vi "HW1_0716007_1011.vi"() -> ()   [LabVIEW 2018]
panel:
  out "Boolean 36":bool
  in  "Boolean 35":bool
  in  "Boolean 30":bool
  out "Boolean 29":bool
  out "Boolean 28":bool
  out "Boolean 27":bool
  out "Boolean 26":bool
  out "Boolean 25":bool
  out "Boolean 24":bool
  out "Boolean 23":bool
  out "Boolean 22":bool
  out "Boolean 21":bool
  out "Boolean 20":bool
  out "Boolean 19":bool
  out "Boolean 18":bool
  out "Boolean 17":bool
  out "Boolean 16":bool
  out "Boolean 15":bool
  out "Boolean 14":bool
  out "Boolean 13":bool
  out "Boolean 12":bool
  out "Boolean 11":bool
  out "Boolean 10":bool
  out "Boolean 9":bool
  out "Boolean 8":bool
  out "Boolean 7":bool
  out "Boolean 6":bool
  out "Boolean 5":bool
  out "Boolean 4":bool
  out "Boolean 3":bool
  out "Boolean 2":bool
  out "two":dbl
  out "History one":dbl
  in  "Boolean":bool
  out "Numeric":dbl
  in  "stop":bool
  out "String 2":string
  out "String":string
  in  "=":bool
  in  "Sqrt":bool
  in  "1/x":bool
  in  "/":bool
  in  "*":bool
  in  "-":bool
  in  "+":bool
  in  ".":bool
  in  "+/-":bool
  in  ")":bool
  in  "(":bool
  in  "Backspace":bool
  in  "C":bool
  in  "CE":bool
  in  "0":bool
  in  "9":bool
  in  "8":bool
  in  "7":bool
  in  "6":bool
  in  "5":bool
  in  "4":bool
  in  "3":bool
  in  "2":bool
  in  "1":bool
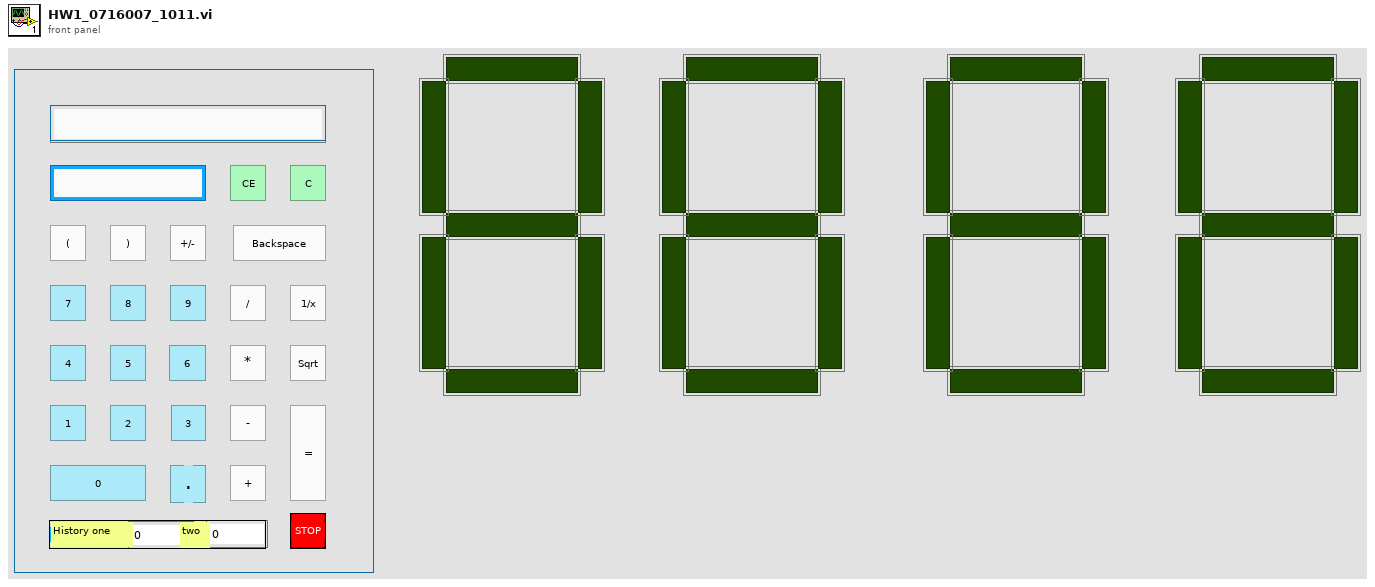
[diagram p1: front panel]
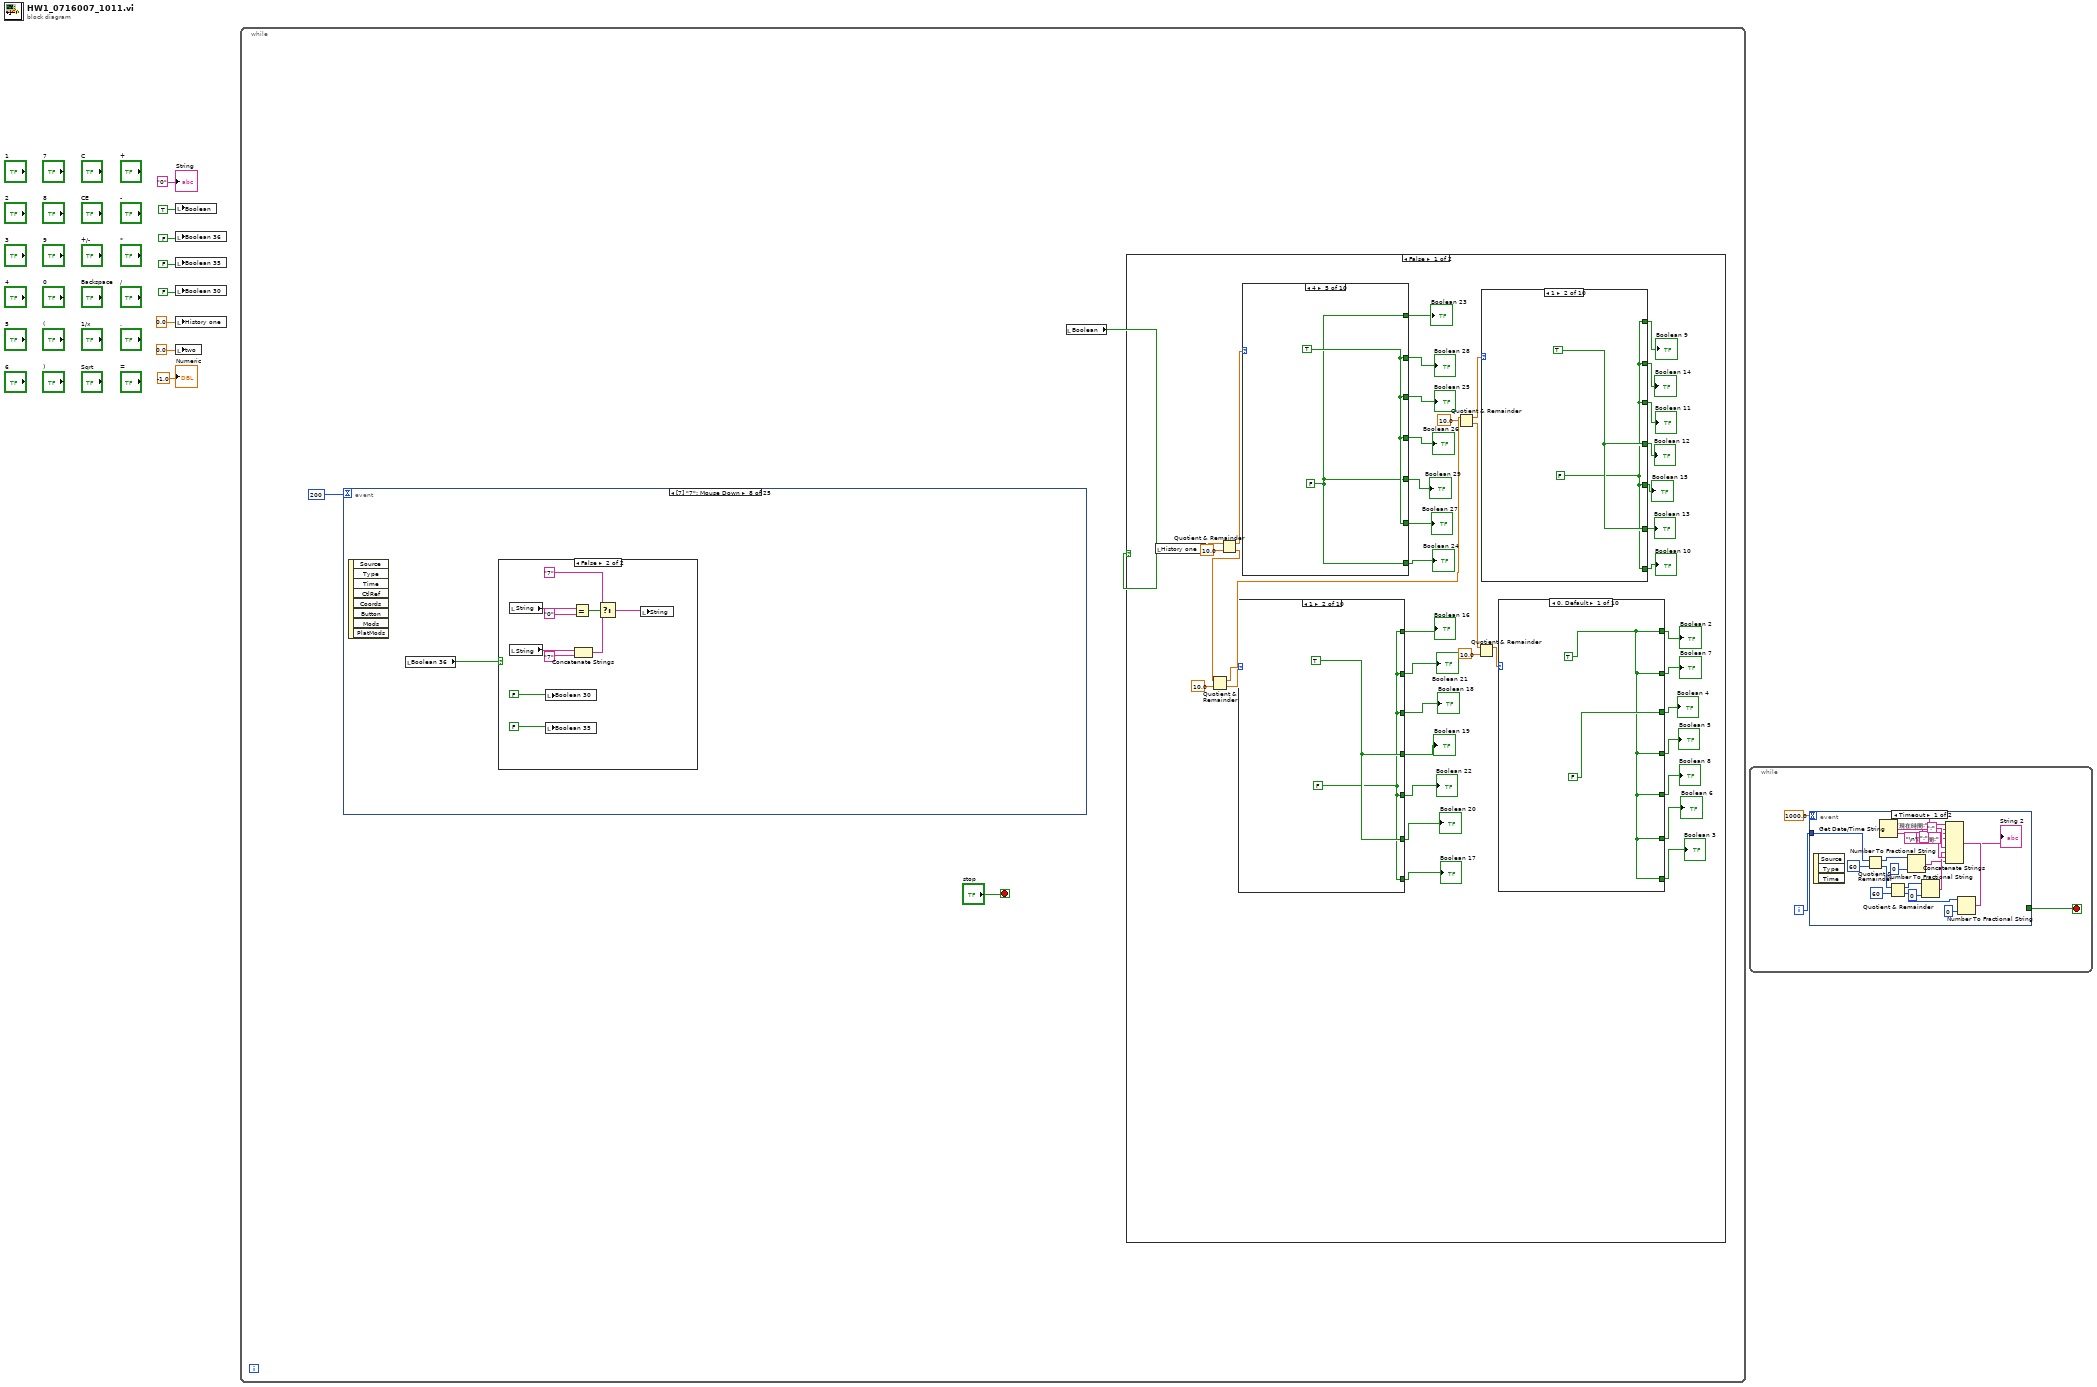
[diagram p0: block diagram]
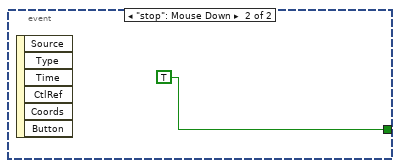
[diagram p2: hidden frame]
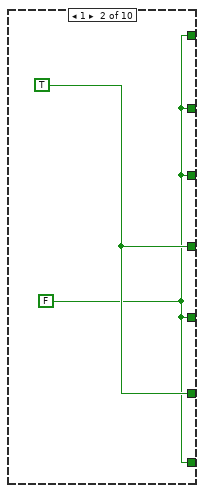
[diagram p3: hidden frame]
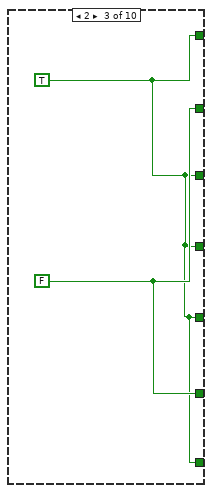
[diagram p4: hidden frame]
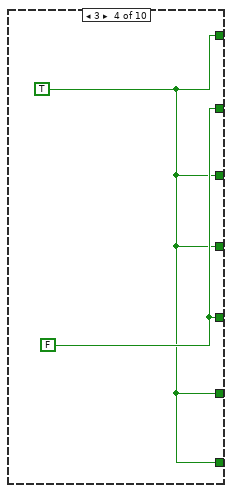
[diagram p5: hidden frame]
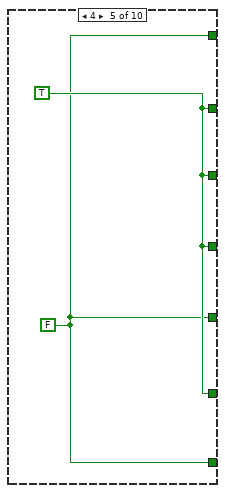
[diagram p6: hidden frame]
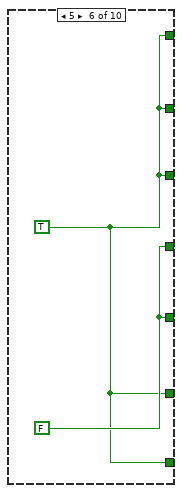
[diagram p7: hidden frame]
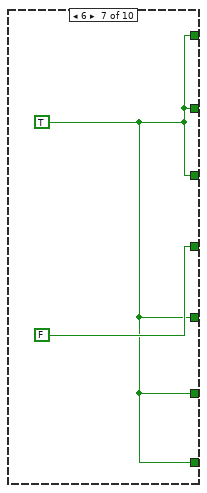
[diagram p8: hidden frame]
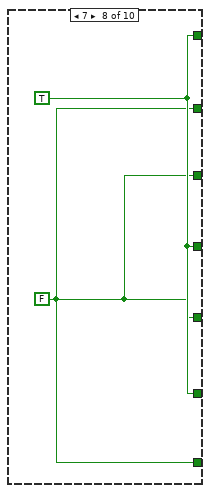
[diagram p9: hidden frame]
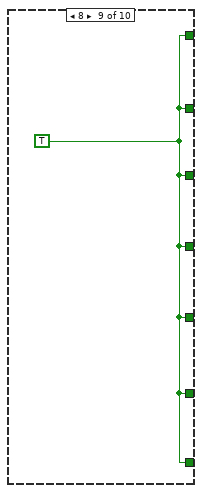
[diagram p10: hidden frame]
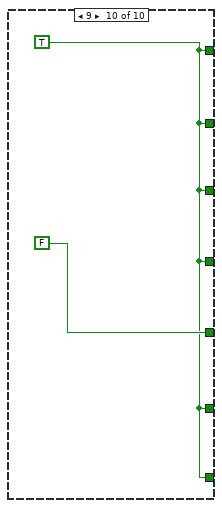
[diagram p11: hidden frame]
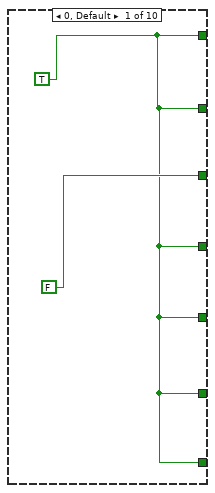
[diagram p12: hidden frame]
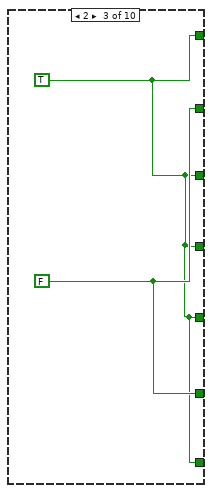
[diagram p13: hidden frame]
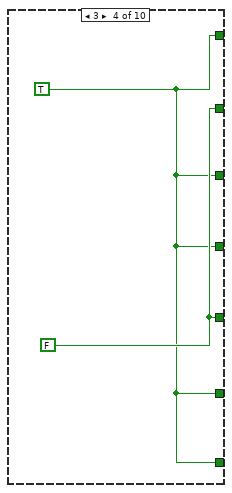
[diagram p14: hidden frame]
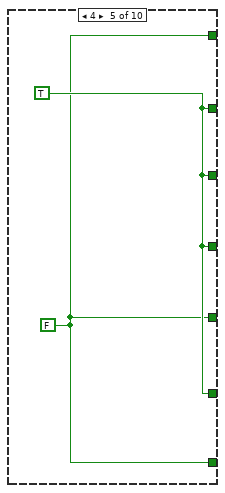
[diagram p15: hidden frame]
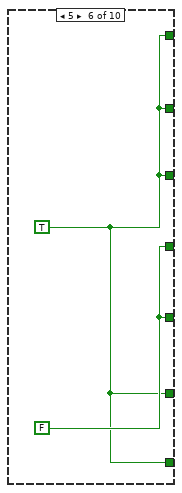
[diagram p16: hidden frame]
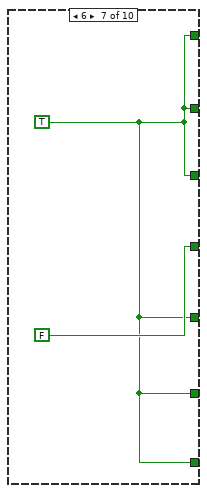
[diagram p17: hidden frame]
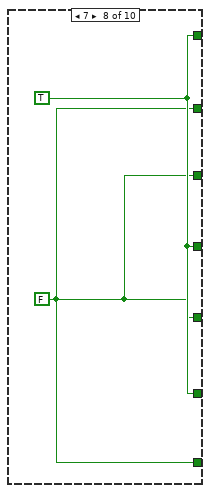
[diagram p18: hidden frame]
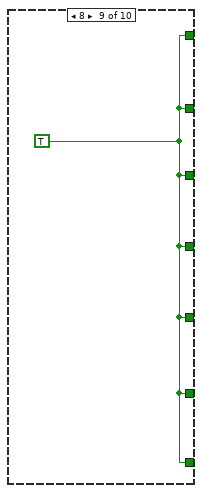
[diagram p19: hidden frame]
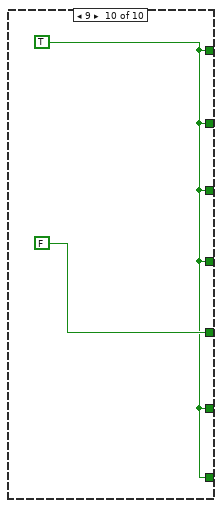
[diagram p20: hidden frame]
diagram:
  n1 = local write "Boolean"(TRUE) -> ()
  n2 = local write "Boolean 36"(FALSE ("Boolean 35")) -> ()
  n3 = local write "Boolean 35"(FALSE ("Boolean 35")) -> ()
  n4 = local write "Boolean 30"(FALSE) -> ()
  n5 = local write "History one"(0.0 ("歷史紀錄2")) -> ()
  n6 = local write "two"(0.0 ("歷史紀錄1")) -> ()
  n7 = while {
    stop <- "stop" stop-if-true
    n8 = event shown="[7] \"7\": Mouse Down" {
      selector: _ -> [_ _ _ _ _ _ _ _ _ _ _ _ _ _ _ _ _ _ _ _ _ _ _ _ _]
      dyn-events: _ -> [_ _ _ _ _ _ _ _ _ _ _ _ _ _ _ _ _ _ _ _ _ _ _ _ _]
      timeout: 200 -> [_ _ _ _ _ _ _ _ _ _ _ _ _ _ _ _ _ _ _ _ _ _ _ _ _]
      event Timeout {
        n9 = event-data() -> ()  [unwired: 1 in, 3 out]
      }
      event "1": Mouse Down {
        n10 = event-data() -> ()  [unwired: 1 in, 8 out]
        n11 = local read "Boolean 10"() -> (w244:bool)
        n12 = case shown="False" w244 {
          frame True {
            n13 = local write "String"("1" ("String")) -> ()
            n14 = local write "Boolean 36"(FALSE) -> ()
            n15 = local write "Boolean 30"(FALSE) -> ()
          }
          frame False {
            n16 = local read "String"() -> (w254:string)
            n17 = local read "String"() -> (w257:string)
            n18 = local write "Boolean 30"(FALSE) -> ()
            n19 = local write "Boolean 35"(FALSE) -> ()
            n20 = Equal?(x=w254, y="0") -> (x = y?=w255:bool)
            n21 = Concatenate Strings(w257, "1" ("string")) -> (w251:string)
            n22 = Select(t="1" ("string"), s=w255, f=w251) -> (s? t:f=w252:string)
            n23 = local write "String"(w252) -> ()
          }
        }
      }
      event "2": Mouse Down {
        n24 = event-data() -> ()  [unwired: 1 in, 8 out]
        n25 = local read "Boolean 36"() -> (w258:bool)
        n26 = case shown="False" w258 {
          frame True {
            n27 = local write "Boolean 36"(FALSE) -> ()
            n28 = local write "String"("2" ("String")) -> ()
            n29 = local write "Boolean 30"(FALSE) -> ()
          }
          frame False {
            n30 = local read "String"() -> (w266:string)
            n31 = local read "String"() -> (w268:string)
            n32 = local write "Boolean 30"(FALSE) -> ()
            n33 = local write "Boolean 35"(FALSE) -> ()
            n34 = Equal?(x=w266, y="0") -> (x = y?=w271:bool)
            n35 = Concatenate Strings(w268, "2" ("string")) -> (w270:string)
            n36 = Select(t="2", s=w271, f=w270) -> (s? t:f=w269:string)
            n37 = local write "String"(w269) -> ()
          }
        }
      }
      event "3": Mouse Down {
        n38 = event-data() -> ()  [unwired: 1 in, 8 out]
        n39 = local read "Boolean 36"() -> (w272:bool)
        n40 = case shown="False" w272 {
          frame True {
            n41 = local write "Boolean 36"(FALSE) -> ()
            n42 = local write "String"("3" ("String")) -> ()
            n43 = local write "Boolean 30"(FALSE) -> ()
          }
          frame False {
            n44 = local read "String"() -> (w280:string)
            n45 = local read "String"() -> (w282:string)
            n46 = local write "Boolean 30"(FALSE) -> ()
            n47 = local write "Boolean 35"(FALSE) -> ()
            n48 = Equal?(x=w280, y="0") -> (x = y?=w285:bool)
            n49 = Concatenate Strings(w282, "3" ("string")) -> (w284:string)
            n50 = Select(t="3", s=w285, f=w284) -> (s? t:f=w283:string)
            n51 = local write "String"(w283) -> ()
          }
        }
      }
      event "4": Mouse Down {
        n52 = event-data() -> ()  [unwired: 1 in, 8 out]
        n53 = local read "Boolean 36"() -> (w286:bool)
        n54 = case shown="False" w286 {
          frame True {
            n55 = local write "Boolean 36"(FALSE) -> ()
            n56 = local write "String"("4" ("String")) -> ()
            n57 = local write "Boolean 30"(FALSE) -> ()
          }
          frame False {
            n58 = local read "String"() -> (w294:string)
            n59 = local read "String"() -> (w296:string)
            n60 = local write "Boolean 30"(FALSE) -> ()
            n61 = local write "Boolean 35"(FALSE) -> ()
            n62 = Equal?(x=w294, y="0") -> (x = y?=w299:bool)
            n63 = Concatenate Strings(w296, "4" ("string")) -> (w298:string)
            n64 = Select(t="4", s=w299, f=w298) -> (s? t:f=w297:string)
            n65 = local write "String"(w297) -> ()
          }
        }
      }
      event "5": Mouse Down {
        n66 = event-data() -> ()  [unwired: 1 in, 8 out]
        n67 = local read "Boolean 36"() -> (w300:bool)
        n68 = case shown="False" w300 {
          frame True {
            n69 = local write "Boolean 36"(FALSE) -> ()
            n70 = local write "String"("5" ("String")) -> ()
            n71 = local write "Boolean 30"(FALSE) -> ()
          }
          frame False {
            n72 = local read "String"() -> (w308:string)
            n73 = local read "String"() -> (w310:string)
            n74 = local write "Boolean 30"(FALSE) -> ()
            n75 = local write "Boolean 35"(FALSE) -> ()
            n76 = Equal?(x=w308, y="0") -> (x = y?=w313:bool)
            n77 = Concatenate Strings(w310, "5" ("string")) -> (w312:string)
            n78 = Select(t="5", s=w313, f=w312) -> (s? t:f=w311:string)
            n79 = local write "String"(w311) -> ()
          }
        }
      }
      event "6": Mouse Down {
        n80 = event-data() -> ()  [unwired: 1 in, 8 out]
        n81 = local read "Boolean 36"() -> (w314:bool)
        n82 = case shown="False" w314 {
          frame True {
            n83 = local write "Boolean 36"(FALSE) -> ()
            n84 = local write "String"("6" ("String")) -> ()
            n85 = local write "Boolean 30"(FALSE) -> ()
          }
          frame False {
            n86 = local read "String"() -> (w322:string)
            n87 = local read "String"() -> (w324:string)
            n88 = local write "Boolean 30"(FALSE) -> ()
            n89 = local write "Boolean 35"(FALSE) -> ()
            n90 = Equal?(x=w322, y="0") -> (x = y?=w327:bool)
            n91 = Concatenate Strings(w324, "6" ("string")) -> (w326:string)
            n92 = Select(t="6", s=w327, f=w326) -> (s? t:f=w325:string)
            n93 = local write "String"(w325) -> ()
          }
        }
      }
      event "7": Mouse Down {
        n94 = event-data() -> ()  [unwired: 1 in, 8 out]
        n95 = local read "Boolean 36"() -> (w328:bool)
        n96 = case shown="False" w328 {
          frame True {
            n97 = local write "Boolean 36"(FALSE) -> ()
            n98 = local write "String"("7" ("String")) -> ()
            n99 = local write "Boolean 30"(FALSE) -> ()
          }
          frame False {
            n100 = local read "String"() -> (w336:string)
            n101 = local read "String"() -> (w338:string)
            n102 = local write "Boolean 30"(FALSE) -> ()
            n103 = local write "Boolean 35"(FALSE) -> ()
            n104 = Equal?(x=w336, y="0") -> (x = y?=w341:bool)
            n105 = Concatenate Strings(w338, "7" ("string")) -> (w340:string)
            n106 = Select(t="7", s=w341, f=w340) -> (s? t:f=w339:string)
            n107 = local write "String"(w339) -> ()
          }
        }
      }
      event "8": Mouse Down {
        n108 = event-data() -> ()  [unwired: 1 in, 8 out]
        n109 = local read "Boolean 36"() -> (w342:bool)
        n110 = case shown="True" w342 {
          frame True {
            n111 = local write "Boolean 36"(FALSE) -> ()
            n112 = local write "String"("8" ("String")) -> ()
            n113 = local write "Boolean 30"(FALSE) -> ()
          }
          frame False {
            n114 = local read "String"() -> (w350:string)
            n115 = local read "String"() -> (w352:string)
            n116 = local write "Boolean 30"(FALSE) -> ()
            n117 = local write "Boolean 35"(FALSE) -> ()
            n118 = Equal?(x=w350, y="0") -> (x = y?=w355:bool)
            n119 = Concatenate Strings(w352, "8" ("string")) -> (w354:string)
            n120 = Select(t="8", s=w355, f=w354) -> (s? t:f=w353:string)
            n121 = local write "String"(w353) -> ()
          }
        }
      }
      event "9": Mouse Down {
        n122 = event-data() -> ()  [unwired: 1 in, 8 out]
        n123 = local read "Boolean 36"() -> (w356:bool)
        n124 = case shown="True" w356 {
          frame True {
            n125 = local write "Boolean 36"(FALSE) -> ()
            n126 = local write "String"("9" ("String")) -> ()
            n127 = local write "Boolean 30"(FALSE) -> ()
          }
          frame False {
            n128 = local read "String"() -> (w364:string)
            n129 = local read "String"() -> (w366:string)
            n130 = local write "Boolean 30"(FALSE) -> ()
            n131 = local write "Boolean 35"(FALSE) -> ()
            n132 = Equal?(x=w364, y="0") -> (x = y?=w369:bool)
            n133 = Concatenate Strings(w366, "9" ("string")) -> (w368:string)
            n134 = Select(t="9", s=w369, f=w368) -> (s? t:f=w367:string)
            n135 = local write "String"(w367) -> ()
          }
        }
      }
      event "0": Mouse Down {
        n136 = event-data() -> ()  [unwired: 1 in, 8 out]
        n137 = local read "Boolean 36"() -> (w370:bool)
        n138 = case shown="True" w370 {
          frame True {
            n139 = local write "Boolean 36"(FALSE) -> ()
            n140 = local write "String"("0" ("String")) -> ()
            n141 = local write "Boolean 30"(FALSE) -> ()
          }
          frame False {
            n142 = local read "String"() -> (w378:string)
            n143 = local read "String"() -> (w380:string)
            n144 = local write "Boolean 30"(FALSE) -> ()
            n145 = local write "Boolean 35"(FALSE) -> ()
            n146 = Equal?(x=w378, y="0") -> (x = y?=w383:bool)
            n147 = Concatenate Strings(w380, "0" ("string")) -> (w382:string)
            n148 = Select(t="0", s=w383, f=w382) -> (s? t:f=w381:string)
            n149 = local write "String"(w381) -> ()
          }
        }
      }
      event "+": Mouse Down {
        n150 = event-data() -> ()  [unwired: 1 in, 8 out]
        n151 = local read "Boolean 36"() -> (w384:bool)
        n152 = case shown="False" w384 {
          frame True {
            n153 = local read "String"() -> (w393:string)
            n154 = local write "Numeric"(1.0 ("Numeric")) -> ()
            n155 = local write "Boolean 30"(TRUE) -> ()
            n156 = local write "Boolean 36"(FALSE) -> ()
            n157 = Search/Split String(string=w393, search string/char (-)="=") -> (match + rest of string=w391:string)  [unwired: 1 in, 2 out]
            n158 = Fract/Exp String To Number(string=w391, offset=1) -> (number=w389:dbl)  [unwired: 2 in, 1 out]
            n159 = Format Into String(format string="%#.6f", w389) -> (resulting string=w394:string)  [unwired: 2 in, 1 out]
            n160 = Concatenate Strings(w394, "+" ("string")) -> (w396:string)
            n161 = local write "String"(w396) -> ()
          }
          frame False {
            n162 = case shown="True" "Boolean 30" {
              tunnel: ["Error" w400] -> w397
              frame True {
              }
              frame False {
                n163 = local read "Numeric"() -> (w402:dbl)
                n164 = case shown="0, Default" w402 {
                  tunnel: [w404 w422 w444 w457 w467 w482] -> w400
                  frame 0, Default {
                    n165 = local read "String"() -> (w406:string)
                    n166 = local write "Numeric"(1.0 ("Numeric")) -> ()
                    n167 = Concatenate Strings(w406, "+" ("string")) -> (w404:string)
                  }
                  frame 1 {
                    n168 = local read "String"() -> (w424:string)
                    n169 = local write "Numeric"(1.0 ("Numeric")) -> ()
                    n170 = Search/Split String(string=w424, search string/char (-)="+") -> (substring before match=w418:string, match + rest of string=w413:string)  [unwired: 1 in, 1 out]
                    n171 = Search/Split String(string=w418, search string/char (-)=".") -> (match + rest of string=w416:string)  [unwired: 1 in, 2 out]
                    n172 = Fract/Exp String To Number(string=w418) -> (number=w425:dbl)  [unwired: 3 in, 1 out]
                    n173 = Fract/Exp String To Number(string=w413, offset=1) -> (number=w426:dbl)  [unwired: 2 in, 1 out]
                    n174 = Search/Split String(string=w413, search string/char (-)=".") -> (match + rest of string=w411:string)  [unwired: 1 in, 2 out]
                    n175 = String Length(string=w416) -> (length=w415:i32)
                    n176 = String Length(string=w411) -> (length=w414:i32)
                    n177 = Decrement(x=w415) -> (x-1=w409:i32)
                    n178 = Add(x=w425, y=w426) -> (x+y=w420:dbl)
                    n179 = Decrement(x=w414) -> (x-1=w408:i32)
                    n180 = Greater?(x=w409, y=w408) -> (0:w410:bool)
                    n181 = Select(t=w409, s=w410, f=w408) -> (s? t:f=w407:i32)
                    n182 = Number To Fractional String(number=w420, precision (6)=w407) -> (F-format string=w419:string)  [unwired: 2 in]
                    n183 = Concatenate Strings(w419, "+" ("string")) -> (w422:string)
                  }
                  frame 2 {
                    n184 = local read "String"() -> (w446:string)
                    n185 = local write "Numeric"(1.0 ("Numeric")) -> ()
                    n186 = Search/Split String(string=w446, search string/char (-)="-") -> (substring before match=w440:string, match + rest of string=w435:string)  [unwired: 1 in, 1 out]
                    n187 = Search/Split String(string=w440, search string/char (-)=".") -> (match + rest of string=w438:string)  [unwired: 1 in, 2 out]
                    n188 = Fract/Exp String To Number(string=w440) -> (number=w447:dbl)  [unwired: 3 in, 1 out]
                    n189 = Fract/Exp String To Number(string=w435, offset=1) -> (number=w448:dbl)  [unwired: 2 in, 1 out]
                    n190 = Search/Split String(string=w435, search string/char (-)=".") -> (match + rest of string=w433:string)  [unwired: 1 in, 2 out]
                    n191 = String Length(string=w438) -> (length=w437:i32)
                    n192 = String Length(string=w433) -> (length=w436:i32)
                    n193 = Decrement(x=w437) -> (x-1=w431:i32)
                    n194 = Subtract(x=w447, y=w448) -> (x-y=w442:dbl)
                    n195 = Decrement(x=w436) -> (x-1=w430:i32)
                    n196 = Greater?(x=w431, y=w430) -> (0:w432:bool)
                    n197 = Select(t=w431, s=w432, f=w430) -> (s? t:f=w429:i32)
                    n198 = Number To Fractional String(number=w442, precision (6)=w429) -> (F-format string=w441:string)  [unwired: 2 in]
                    n199 = Concatenate Strings(w441, "+" ("string")) -> (w444:string)
                  }
                  frame 3 {
                    n200 = local read "String"() -> (w459:string)
                    n201 = local write "Numeric"(1.0 ("Numeric")) -> ()
                    n202 = Search/Split String(string=w459, search string/char (-)="*") -> (substring before match=w455:string, match + rest of string=w454:string)  [unwired: 1 in, 1 out]
                    n203 = Fract/Exp String To Number(string=w454, offset=1) -> (number=w461:dbl)  [unwired: 2 in, 1 out]
                    n204 = Fract/Exp String To Number(string=w455) -> (number=w460:dbl)  [unwired: 3 in, 1 out]
                    n205 = Multiply(x=w460, y=w461) -> (x*y=w453:dbl)
                    n206 = Format Into String(format string="%#.6f", w453) -> (resulting string=w451:string)  [unwired: 2 in, 1 out]
                    n207 = Concatenate Strings(w451, "+" ("string")) -> (w457:string)
                  }
                  frame 4 {
                    n208 = local read "String"() -> (w476:string)
                    n209 = local write "Numeric"(1.0 ("Numeric")) -> ()
                    n210 = Search/Split String(string=w476, search string/char (-)="/") -> (substring before match=w473:string, match + rest of string=w472:string)  [unwired: 1 in, 1 out]
                    n211 = Fract/Exp String To Number(string=w473) -> (number=w477:dbl)  [unwired: 3 in, 1 out]
                    n212 = Fract/Exp String To Number(string=w472, offset=1) -> (number=w471:dbl)  [unwired: 2 in, 1 out]
                    n213 = Equal To 0?(x=w471) -> (x = 0?=w470:bool)
                    n214 = Divide(x=w477, y=w471) -> (x/y=w466:dbl)
                    n215 = Format Into String(format string="%#.6f", w466) -> (resulting string=w464:string)  [unwired: 2 in, 1 out]
                    n216 = Concatenate Strings(w464, "+" ("string")) -> (w468:string)
                    n217 = Select(t="Error", s=w470, f=w468) -> (s? t:f=w467:string)
                  }
                  frame 5 {
                    n218 = local read "String"() -> (w480:string)
                    n219 = local write "Numeric"(1.0 ("Numeric")) -> ()
                    n220 = Concatenate Strings(w480, "+" ("string")) -> (w482:string)
                  }
                }
                n221 = local write "Boolean 30"(TRUE) -> ()
              }
            }
            n222 = local write "String"(w397) -> ()
          }
        }
      }
      event "1/x": Mouse Down {
        n223 = event-data() -> ()  [unwired: 1 in, 8 out]
        n224 = local read "Numeric"() -> (w484:dbl)
        n225 = case shown="1" w484 {
          tunnel: [w486 w492 w506 w516 w528] -> w485
          frame 0, Default {
            n226 = local read "String"() -> (w490:string)
            n227 = Fract/Exp String To Number(string=w490) -> (number=w489:dbl)  [unwired: 3 in, 1 out]
            n228 = local write "Numeric"(1.0 ("Numeric")) -> ()
            n229 = Reciprocal(x=w489) -> (1/x=w487:dbl)
            n230 = Format Into String(format string="%#.6f", w487) -> (resulting string=w486:string)  [unwired: 2 in, 1 out]
          }
          frame 1 {
            n231 = local read "String"() -> (w499:string)
            n232 = local write "Numeric"(-1.0 ("Numeric")) -> ()
            n233 = Search/Split String(string=w499, search string/char (-)="+") -> (substring before match=w497:string, match + rest of string=w496:string)  [unwired: 1 in, 1 out]
            n234 = Fract/Exp String To Number(string=w497) -> (number=w500:dbl)  [unwired: 3 in, 1 out]
            n235 = Fract/Exp String To Number(string=w496, offset=1) -> (number=w501:dbl)  [unwired: 2 in, 1 out]
            n236 = Add(x=w500, y=w501) -> (x+y=w495:dbl)
            n237 = Reciprocal(x=w495) -> (1/x=w493:dbl)
            n238 = Format Into String(format string="%#.6f", w493) -> (resulting string=w492:string)  [unwired: 2 in, 1 out]
          }
          frame 2 {
            n239 = local read "String"() -> (w511:string)
            n240 = local write "Numeric"(-1.0 ("Numeric")) -> ()
            n241 = Search/Split String(string=w511, search string/char (-)="-") -> (substring before match=w509:string, match + rest of string=w508:string)  [unwired: 1 in, 1 out]
            n242 = Fract/Exp String To Number(string=w509) -> (number=w512:dbl)  [unwired: 3 in, 1 out]
            n243 = Fract/Exp String To Number(string=w508, offset=1) -> (number=w513:dbl)  [unwired: 2 in, 1 out]
            n244 = Subtract(x=w512, y=w513) -> (x-y=w507:dbl)
            n245 = Reciprocal(x=w507) -> (1/x=w505:dbl)
            n246 = Format Into String(format string="%#.6f", w505) -> (resulting string=w506:string)  [unwired: 2 in, 1 out]
          }
          frame 3 {
            n247 = local read "String"() -> (w523:string)
            n248 = local write "Numeric"(-1.0 ("Numeric")) -> ()
            n249 = Search/Split String(string=w523, search string/char (-)="*") -> (substring before match=w521:string, match + rest of string=w520:string)  [unwired: 1 in, 1 out]
            n250 = Fract/Exp String To Number(string=w521) -> (number=w524:dbl)  [unwired: 3 in, 1 out]
            n251 = Fract/Exp String To Number(string=w520, offset=1) -> (number=w525:dbl)  [unwired: 2 in, 1 out]
            n252 = Multiply(x=w524, y=w525) -> (x*y=w519:dbl)
            n253 = Reciprocal(x=w519) -> (1/x=w517:dbl)
            n254 = Format Into String(format string="%#.6f", w517) -> (resulting string=w516:string)  [unwired: 2 in, 1 out]
          }
          frame 4 {
            n255 = local read "String"() -> (w536:string)
            n256 = local write "Numeric"(-1.0 ("Numeric")) -> ()
            n257 = Search/Split String(string=w536, search string/char (-)="/") -> (substring before match=w538:string, match + rest of string=w539:string)  [unwired: 1 in, 1 out]
            n258 = Fract/Exp String To Number(string=w538) -> (number=w535:dbl)  [unwired: 3 in, 1 out]
            n259 = Fract/Exp String To Number(string=w539, offset=1) -> (number=w534:dbl)  [unwired: 2 in, 1 out]
            n260 = Divide(x=w535, y=w534) -> (x/y=w531:dbl)
            n261 = Reciprocal(x=w531) -> (1/x=w529:dbl)
            n262 = Format Into String(format string="%#.6f", w529) -> (resulting string=w528:string)  [unwired: 2 in, 1 out]
          }
        }
        n263 = local write "String"(w485) -> ()
      }
      event "Sqrt": Mouse Down {
        n264 = event-data() -> ()  [unwired: 1 in, 8 out]
        n265 = local read "Numeric"() -> (w540:dbl)
        n266 = case shown="0, Default" w540 {
          tunnel: [w542 w548 w562 w572 w584] -> w541
          frame 0, Default {
            n267 = local read "String"() -> (w546:string)
            n268 = local write "Numeric"(1.0 ("Numeric")) -> ()
            n269 = Fract/Exp String To Number(string=w546) -> (number=w545:dbl)  [unwired: 3 in, 1 out]
            n270 = Square Root(x=w545) -> (sqrt(x)=w543:dbl)
            n271 = Format Into String(format string="%#.6f", w543) -> (resulting string=w542:string)  [unwired: 2 in, 1 out]
          }
          frame 1 {
            n272 = local read "String"() -> (w555:string)
            n273 = local write "Numeric"(-1.0 ("Numeric")) -> ()
            n274 = Search/Split String(string=w555, search string/char (-)="+") -> (substring before match=w553:string, match + rest of string=w552:string)  [unwired: 1 in, 1 out]
            n275 = Fract/Exp String To Number(string=w553) -> (number=w556:dbl)  [unwired: 3 in, 1 out]
            n276 = Fract/Exp String To Number(string=w552, offset=1) -> (number=w557:dbl)  [unwired: 2 in, 1 out]
            n277 = Add(x=w556, y=w557) -> (x+y=w551:dbl)
            n278 = Square Root(x=w551) -> (sqrt(x)=w549:dbl)
            n279 = Format Into String(format string="%#.6f", w549) -> (resulting string=w548:string)  [unwired: 2 in, 1 out]
          }
          frame 2 {
            n280 = local read "String"() -> (w567:string)
            n281 = local write "Numeric"(-1.0 ("Numeric")) -> ()
            n282 = Search/Split String(string=w567, search string/char (-)="-") -> (substring before match=w565:string, match + rest of string=w564:string)  [unwired: 1 in, 1 out]
            n283 = Fract/Exp String To Number(string=w565) -> (number=w568:dbl)  [unwired: 3 in, 1 out]
            n284 = Fract/Exp String To Number(string=w564, offset=1) -> (number=w569:dbl)  [unwired: 2 in, 1 out]
            n285 = Subtract(x=w568, y=w569) -> (x-y=w563:dbl)
            n286 = Square Root(x=w563) -> (sqrt(x)=w561:dbl)
            n287 = Format Into String(format string="%#.6f", w561) -> (resulting string=w562:string)  [unwired: 2 in, 1 out]
          }
          frame 3 {
            n288 = local read "String"() -> (w579:string)
            n289 = local write "Numeric"(-1.0 ("Numeric")) -> ()
            n290 = Search/Split String(string=w579, search string/char (-)="*") -> (substring before match=w577:string, match + rest of string=w576:string)  [unwired: 1 in, 1 out]
            n291 = Fract/Exp String To Number(string=w577) -> (number=w580:dbl)  [unwired: 3 in, 1 out]
            n292 = Fract/Exp String To Number(string=w576, offset=1) -> (number=w581:dbl)  [unwired: 2 in, 1 out]
            n293 = Multiply(x=w580, y=w581) -> (x*y=w575:dbl)
            n294 = Square Root(x=w575) -> (sqrt(x)=w573:dbl)
            n295 = Format Into String(format string="%#.6f", w573) -> (resulting string=w572:string)  [unwired: 2 in, 1 out]
          }
          frame 4 {
            n296 = local read "String"() -> (w592:string)
            n297 = local write "Numeric"(-1.0 ("Numeric")) -> ()
            n298 = Search/Split String(string=w592, search string/char (-)="/") -> (substring before match=w594:string, match + rest of string=w595:string)  [unwired: 1 in, 1 out]
            n299 = Fract/Exp String To Number(string=w594) -> (number=w591:dbl)  [unwired: 3 in, 1 out]
            n300 = Fract/Exp String To Number(string=w595, offset=1) -> (number=w590:dbl)  [unwired: 2 in, 1 out]
            n301 = Divide(x=w591, y=w590) -> (x/y=w587:dbl)
            n302 = Square Root(x=w587) -> (sqrt(x)=w585:dbl)
            n303 = Format Into String(format string="%#.6f", w585) -> (resulting string=w584:string)  [unwired: 2 in, 1 out]
          }
        }
        n304 = local write "String"(w541) -> ()
      }
      event "CE": Mouse Down {
        n305 = event-data() -> ()  [unwired: 1 in, 8 out]
        n306 = local read "String"() -> (w596:string)
        n307 = case shown="\"True\", Default" w596 {
          frame "Error" {
            n308 = local write "String"("0" ("String")) -> ()
          }
          frame "True", Default {
            n309 = local read "Numeric"() -> (w599:dbl)
            n310 = case shown="1" w599 {
              tunnel: ["0" w602 w607 w612 w617] -> w598
              frame 0, Default {
              }
              frame 1 {
                n311 = local read "String"() -> (w604:string)
                n312 = Search/Split String(string=w604, search string/char (-)="+") -> (substring before match=w601:string)  [unwired: 1 in, 2 out]
                n313 = Concatenate Strings(w601, "+" ("string")) -> (w602:string)
              }
              frame 2 {
                n314 = local read "String"() -> (w609:string)
                n315 = Search/Split String(string=w609, search string/char (-)="-") -> (substring before match=w606:string)  [unwired: 1 in, 2 out]
                n316 = Concatenate Strings(w606, "-" ("string")) -> (w607:string)
              }
              frame 3 {
                n317 = local read "String"() -> (w614:string)
                n318 = Search/Split String(string=w614, search string/char (-)="*") -> (substring before match=w611:string)  [unwired: 1 in, 2 out]
                n319 = Concatenate Strings(w611, "*" ("string")) -> (w612:string)
              }
              frame 4 {
                n320 = local read "String"() -> (w619:string)
                n321 = Search/Split String(string=w619, search string/char (-)="/") -> (substring before match=w616:string)  [unwired: 1 in, 2 out]
                n322 = Concatenate Strings(w616, "/" ("string")) -> (w617:string)
              }
            }
            n323 = local write "String"(w598) -> ()
          }
        }
      }
      event "-": Mouse Down {
        n324 = event-data() -> ()  [unwired: 1 in, 8 out]
        n325 = local read "Boolean 36"() -> (w621:bool)
        n326 = case shown="True" w621 {
          frame True {
            n327 = local read "String"() -> (w630:string)
            n328 = local write "Boolean 30"(TRUE) -> ()
            n329 = local write "Numeric"(2.0 ("Numeric")) -> ()
            n330 = local write "Boolean 36"(FALSE) -> ()
            n331 = Search/Split String(string=w630, search string/char (-)="=") -> (match + rest of string=w628:string)  [unwired: 1 in, 2 out]
            n332 = Fract/Exp String To Number(string=w628, offset=1) -> (number=w626:dbl)  [unwired: 2 in, 1 out]
            n333 = Format Into String(format string="%#.6f", w626) -> (resulting string=w631:string)  [unwired: 2 in, 1 out]
            n334 = Concatenate Strings(w631, "-" ("string")) -> (w633:string)
            n335 = local write "String"(w633) -> ()
          }
          frame False {
            n336 = local read "Boolean 30"() -> (w635:bool)
            n337 = case shown="False" w635 {
              tunnel: ["Error" w637] -> w634
              frame True {
              }
              frame False {
                n338 = local read "Numeric"() -> (w639:dbl)
                n339 = case shown="2" w639 {
                  tunnel: [w641 w659 w681 w694 w706 w718] -> w637
                  frame 0, Default {
                    n340 = local read "String"() -> (w643:string)
                    n341 = local write "Numeric"(2.0 ("Numeric")) -> ()
                    n342 = Concatenate Strings(w643, "-" ("string")) -> (w641:string)
                  }
                  frame 1 {
                    n343 = local read "String"() -> (w661:string)
                    n344 = local write "Numeric"(2.0 ("Numeric")) -> ()
                    n345 = Search/Split String(string=w661, search string/char (-)="+") -> (substring before match=w655:string, match + rest of string=w650:string)  [unwired: 1 in, 1 out]
                    n346 = Search/Split String(string=w655, search string/char (-)=".") -> (match + rest of string=w653:string)  [unwired: 1 in, 2 out]
                    n347 = Search/Split String(string=w650, search string/char (-)=".") -> (match + rest of string=w648:string)  [unwired: 1 in, 2 out]
                    n348 = Fract/Exp String To Number(string=w655) -> (number=w662:dbl)  [unwired: 3 in, 1 out]
                    n349 = Fract/Exp String To Number(string=w650, offset=1) -> (number=w663:dbl)  [unwired: 2 in, 1 out]
                    n350 = String Length(string=w653) -> (length=w652:i32)
                    n351 = String Length(string=w648) -> (length=w651:i32)
                    n352 = Add(x=w662, y=w663) -> (x+y=w657:dbl)
                    n353 = Decrement(x=w652) -> (x-1=w646:i32)
                    n354 = Decrement(x=w651) -> (x-1=w645:i32)
                    n355 = Greater?(x=w646, y=w645) -> (0:w647:bool)
                    n356 = Select(t=w646, s=w647, f=w645) -> (s? t:f=w644:i32)
                    n357 = Number To Fractional String(number=w657, precision (6)=w644) -> (F-format string=w656:string)  [unwired: 2 in]
                    n358 = Concatenate Strings(w656, "-" ("string")) -> (w659:string)
                  }
                  frame 2 {
                    n359 = local read "String"() -> (w683:string)
                    n360 = local write "Numeric"(2.0 ("Numeric")) -> ()
                    n361 = Search/Split String(string=w683, search string/char (-)="-") -> (substring before match=w677:string, match + rest of string=w672:string)  [unwired: 1 in, 1 out]
                    n362 = Search/Split String(string=w677, search string/char (-)=".") -> (match + rest of string=w675:string)  [unwired: 1 in, 2 out]
                    n363 = Search/Split String(string=w672, search string/char (-)=".") -> (match + rest of string=w670:string)  [unwired: 1 in, 2 out]
                    n364 = Fract/Exp String To Number(string=w677) -> (number=w684:dbl)  [unwired: 3 in, 1 out]
                    n365 = Fract/Exp String To Number(string=w672, offset=1) -> (number=w685:dbl)  [unwired: 2 in, 1 out]
                    n366 = String Length(string=w675) -> (length=w674:i32)
                    n367 = String Length(string=w670) -> (length=w673:i32)
                    n368 = Subtract(x=w684, y=w685) -> (x-y=w679:dbl)
                    n369 = Decrement(x=w674) -> (x-1=w668:i32)
                    n370 = Decrement(x=w673) -> (x-1=w667:i32)
                    n371 = Greater?(x=w668, y=w667) -> (0:w669:bool)
                    n372 = Select(t=w668, s=w669, f=w667) -> (s? t:f=w666:i32)
                    n373 = Number To Fractional String(number=w679, precision (6)=w666) -> (F-format string=w678:string)  [unwired: 2 in]
                    n374 = Concatenate Strings(w678, "-" ("string")) -> (w681:string)
                  }
                  frame 3 {
                    n375 = local read "String"() -> (w696:string)
                    n376 = Search/Split String(string=w696, search string/char (-)="*") -> (substring before match=w692:string, match + rest of string=w691:string)  [unwired: 1 in, 1 out]
                    n377 = Fract/Exp String To Number(string=w692) -> (number=w697:dbl)  [unwired: 3 in, 1 out]
                    n378 = Fract/Exp String To Number(string=w691, offset=1) -> (number=w698:dbl)  [unwired: 2 in, 1 out]
                    n379 = local write "Numeric"(2.0 ("Numeric")) -> ()
                    n380 = Multiply(x=w697, y=w698) -> (x*y=w689:dbl)
                    n381 = Format Into String(format string="%#.6f", w689) -> (resulting string=w688:string)  [unwired: 2 in, 1 out]
                    n382 = Concatenate Strings(w688, "-" ("string")) -> (w694:string)
                  }
                  frame 4 {
                    n383 = local read "String"() -> (w712:string)
                    n384 = local write "Numeric"(2.0 ("Numeric")) -> ()
                    n385 = Search/Split String(string=w712, search string/char (-)="/") -> (substring before match=w710:string, match + rest of string=w709:string)  [unwired: 1 in, 1 out]
                    n386 = Fract/Exp String To Number(string=w710) -> (number=w713:dbl)  [unwired: 3 in, 1 out]
                    n387 = Fract/Exp String To Number(string=w709, offset=1) -> (number=w708:dbl)  [unwired: 2 in, 1 out]
                    n388 = Divide(x=w713, y=w708) -> (x/y=w702:dbl)
                    n389 = Equal To 0?(x=w708) -> (x = 0?=w707:bool)
                    n390 = Format Into String(format string="%#.6f", w702) -> (resulting string=w701:string)  [unwired: 2 in, 1 out]
                    n391 = Concatenate Strings(w701, "-" ("string")) -> (w705:string)
                    n392 = Select(t="Error", s=w707, f=w705) -> (s? t:f=w706:string)
                  }
                  frame 5 {
                    n393 = local write "Numeric"(2.0 ("Numeric")) -> ()
                    n394 = local read "String"() -> (w717:string)
                    n395 = Concatenate Strings(w717, "-" ("string")) -> (w718:string)
                  }
                }
                n396 = local write "Boolean 30"(TRUE) -> ()
              }
            }
            n397 = local write "String"(w634) -> ()
          }
        }
      }
      event "*": Mouse Down {
        n398 = event-data() -> ()  [unwired: 1 in, 8 out]
        n399 = local read "Boolean 36"() -> (w721:bool)
        n400 = case shown="True" w721 {
          frame True {
            n401 = local write "Numeric"(3.0 ("Numeric")) -> ()
            n402 = local read "String"() -> (w728:string)
            n403 = local write "Boolean 30"(TRUE) -> ()
            n404 = local write "Boolean 36"(FALSE) -> ()
            n405 = Search/Split String(string=w728, search string/char (-)="=") -> (match + rest of string=w726:string)  [unwired: 1 in, 2 out]
            n406 = Fract/Exp String To Number(string=w726, offset=1) -> (number=w724:dbl)  [unwired: 2 in, 1 out]
            n407 = Format Into String(format string="%#.6f", w724) -> (resulting string=w729:string)  [unwired: 2 in, 1 out]
            n408 = Concatenate Strings(w729, "*" ("string")) -> (w731:string)
            n409 = local write "String"(w731) -> ()
          }
          frame False {
            n410 = local read "Boolean 30"() -> (w734:bool)
            n411 = case shown="True" w734 {
              tunnel: ["Error" w739] -> w735
              frame True {
              }
              frame False {
                n412 = local read "Numeric"() -> (w738:dbl)
                n413 = case shown="4" w738 {
                  tunnel: [w741 w759 w781 w794 w805 w818] -> w739
                  frame 0, Default {
                    n414 = local read "String"() -> (w743:string)
                    n415 = Concatenate Strings(w743, "*" ("string")) -> (w741:string)
                    n416 = local write "Numeric"(3.0 ("Numeric")) -> ()
                  }
                  frame 1 {
                    n417 = local read "String"() -> (w761:string)
                    n418 = Search/Split String(string=w761, search string/char (-)="+") -> (substring before match=w755:string, match + rest of string=w750:string)  [unwired: 1 in, 1 out]
                    n419 = Search/Split String(string=w755, search string/char (-)=".") -> (match + rest of string=w753:string)  [unwired: 1 in, 2 out]
                    n420 = Search/Split String(string=w750, search string/char (-)=".") -> (match + rest of string=w748:string)  [unwired: 1 in, 2 out]
                    n421 = Fract/Exp String To Number(string=w755) -> (number=w762:dbl)  [unwired: 3 in, 1 out]
                    n422 = Fract/Exp String To Number(string=w750, offset=1) -> (number=w763:dbl)  [unwired: 2 in, 1 out]
                    n423 = String Length(string=w753) -> (length=w752:i32)
                    n424 = String Length(string=w748) -> (length=w751:i32)
                    n425 = local write "Numeric"(3.0 ("Numeric")) -> ()
                    n426 = Add(x=w762, y=w763) -> (x+y=w757:dbl)
                    n427 = Decrement(x=w752) -> (x-1=w746:i32)
                    n428 = Decrement(x=w751) -> (x-1=w745:i32)
                    n429 = Greater?(x=w746, y=w745) -> (0:w747:bool)
                    n430 = Select(t=w746, s=w747, f=w745) -> (s? t:f=w744:i32)
                    n431 = Number To Fractional String(number=w757, precision (6)=w744) -> (F-format string=w756:string)  [unwired: 2 in]
                    n432 = Concatenate Strings(w756, "*" ("string")) -> (w759:string)
                  }
                  frame 2 {
                    n433 = local read "String"() -> (w783:string)
                    n434 = local write "Numeric"(3.0 ("Numeric")) -> ()
                    n435 = Search/Split String(string=w783, search string/char (-)="-") -> (substring before match=w777:string, match + rest of string=w772:string)  [unwired: 1 in, 1 out]
                    n436 = Search/Split String(string=w777, search string/char (-)=".") -> (match + rest of string=w775:string)  [unwired: 1 in, 2 out]
                    n437 = Search/Split String(string=w772, search string/char (-)=".") -> (match + rest of string=w770:string)  [unwired: 1 in, 2 out]
                    n438 = Fract/Exp String To Number(string=w777) -> (number=w784:dbl)  [unwired: 3 in, 1 out]
                    n439 = Fract/Exp String To Number(string=w772, offset=1) -> (number=w785:dbl)  [unwired: 2 in, 1 out]
                    n440 = String Length(string=w775) -> (length=w774:i32)
                    n441 = String Length(string=w770) -> (length=w773:i32)
                    n442 = Subtract(x=w784, y=w785) -> (x-y=w779:dbl)
                    n443 = Decrement(x=w774) -> (x-1=w768:i32)
                    n444 = Decrement(x=w773) -> (x-1=w767:i32)
                    n445 = Greater?(x=w768, y=w767) -> (0:w769:bool)
                    n446 = Select(t=w768, s=w769, f=w767) -> (s? t:f=w766:i32)
                    n447 = Number To Fractional String(number=w779, precision (6)=w766) -> (F-format string=w778:string)  [unwired: 2 in]
                    n448 = Concatenate Strings(w778, "*" ("string")) -> (w781:string)
                  }
                  frame 3 {
                    n449 = local read "String"() -> (w796:string)
                    n450 = local write "Numeric"(3.0 ("Numeric")) -> ()
                    n451 = Search/Split String(string=w796, search string/char (-)="*") -> (substring before match=w792:string, match + rest of string=w791:string)  [unwired: 1 in, 1 out]
                    n452 = Fract/Exp String To Number(string=w792) -> (number=w797:dbl)  [unwired: 3 in, 1 out]
                    n453 = Fract/Exp String To Number(string=w791, offset=1) -> (number=w798:dbl)  [unwired: 2 in, 1 out]
                    n454 = Multiply(x=w797, y=w798) -> (x*y=w789:dbl)
                    n455 = Format Into String(format string="%#.6f", w789) -> (resulting string=w788:string)  [unwired: 2 in, 1 out]
                    n456 = Concatenate Strings(w788, "*" ("string")) -> (w794:string)
                  }
                  frame 4 {
                    n457 = local read "String"() -> (w812:string)
                    n458 = local write "Numeric"(3.0 ("Numeric")) -> ()
                    n459 = Search/Split String(string=w812, search string/char (-)="/") -> (substring before match=w810:string, match + rest of string=w809:string)  [unwired: 1 in, 1 out]
                    n460 = Fract/Exp String To Number(string=w810) -> (number=w813:dbl)  [unwired: 3 in, 1 out]
                    n461 = Fract/Exp String To Number(string=w809, offset=1) -> (number=w808:dbl)  [unwired: 2 in, 1 out]
                    n462 = Equal To 0?(x=w808) -> (x = 0?=w807:bool)
                    n463 = Divide(x=w813, y=w808) -> (x/y=w802:dbl)
                    n464 = Format Into String(format string="%#.6f", w802) -> (resulting string=w801:string)  [unwired: 2 in, 1 out]
                    n465 = Concatenate Strings(w801, "*" ("string")) -> (w806:string)
                    n466 = Select(t="Error", s=w807, f=w806) -> (s? t:f=w805:string)
                  }
                  frame 5 {
                    n467 = local read "String"() -> (w817:string)
                    n468 = local write "Numeric"(3.0 ("Numeric")) -> ()
                    n469 = Concatenate Strings(w817, "*" ("string")) -> (w818:string)
                  }
                }
                n470 = local write "Boolean 30"(TRUE) -> ()
              }
            }
            n471 = local write "String"(w735) -> ()
          }
        }
      }
      event "/": Mouse Down {
        n472 = event-data() -> ()  [unwired: 1 in, 8 out]
        n473 = local read "Boolean 36"() -> (w821:bool)
        n474 = case shown="True" w821 {
          frame True {
            n475 = local write "Numeric"(4.0 ("Numeric")) -> ()
            n476 = local read "String"() -> (w828:string)
            n477 = local write "Boolean 30"(TRUE) -> ()
            n478 = local write "Boolean 36"(FALSE) -> ()
            n479 = Search/Split String(string=w828, search string/char (-)="=") -> (match + rest of string=w826:string)  [unwired: 1 in, 2 out]
            n480 = Fract/Exp String To Number(string=w826, offset=1) -> (number=w824:dbl)  [unwired: 2 in, 1 out]
            n481 = Format Into String(format string="%#.6f", w824) -> (resulting string=w829:string)  [unwired: 2 in, 1 out]
            n482 = Concatenate Strings(w829, "/" ("string")) -> (w831:string)
            n483 = local write "String"(w831) -> ()
          }
          frame False {
            n484 = local read "Boolean 30"() -> (w834:bool)
            n485 = case shown="False" w834 {
              tunnel: ["Error" w839] -> w835
              frame True {
              }
              frame False {
                n486 = local read "Numeric"() -> (w838:dbl)
                n487 = case shown="5" w838 {
                  tunnel: [w841 w859 w881 w894 w904 w919] -> w839
                  frame 0, Default {
                    n488 = local read "String"() -> (w843:string)
                    n489 = local write "Numeric"(4.0 ("Numeric")) -> ()
                    n490 = Concatenate Strings(w843, "/" ("string")) -> (w841:string)
                  }
                  frame 1 {
                    n491 = local read "String"() -> (w861:string)
                    n492 = local write "Numeric"(4.0 ("Numeric")) -> ()
                    n493 = Search/Split String(string=w861, search string/char (-)="+") -> (substring before match=w855:string, match + rest of string=w850:string)  [unwired: 1 in, 1 out]
                    n494 = Search/Split String(string=w855, search string/char (-)=".") -> (match + rest of string=w853:string)  [unwired: 1 in, 2 out]
                    n495 = Search/Split String(string=w850, search string/char (-)=".") -> (match + rest of string=w848:string)  [unwired: 1 in, 2 out]
                    n496 = Fract/Exp String To Number(string=w855) -> (number=w862:dbl)  [unwired: 3 in, 1 out]
                    n497 = Fract/Exp String To Number(string=w850, offset=1) -> (number=w863:dbl)  [unwired: 2 in, 1 out]
                    n498 = String Length(string=w853) -> (length=w852:i32)
                    n499 = String Length(string=w848) -> (length=w851:i32)
                    n500 = Add(x=w862, y=w863) -> (x+y=w857:dbl)
                    n501 = Decrement(x=w852) -> (x-1=w846:i32)
                    n502 = Decrement(x=w851) -> (x-1=w845:i32)
                    n503 = Greater?(x=w846, y=w845) -> (0:w847:bool)
                    n504 = Select(t=w846, s=w847, f=w845) -> (s? t:f=w844:i32)
                    n505 = Number To Fractional String(number=w857, precision (6)=w844) -> (F-format string=w856:string)  [unwired: 2 in]
                    n506 = Concatenate Strings(w856, "/" ("string")) -> (w859:string)
                  }
                  frame 2 {
                    n507 = local read "String"() -> (w883:string)
                    n508 = local write "Numeric"(4.0 ("Numeric")) -> ()
                    n509 = Search/Split String(string=w883, search string/char (-)="-") -> (substring before match=w877:string, match + rest of string=w872:string)  [unwired: 1 in, 1 out]
                    n510 = Search/Split String(string=w877, search string/char (-)=".") -> (match + rest of string=w875:string)  [unwired: 1 in, 2 out]
                    n511 = Search/Split String(string=w872, search string/char (-)=".") -> (match + rest of string=w870:string)  [unwired: 1 in, 2 out]
                    n512 = Fract/Exp String To Number(string=w877) -> (number=w884:dbl)  [unwired: 3 in, 1 out]
                    n513 = Fract/Exp String To Number(string=w872, offset=1) -> (number=w885:dbl)  [unwired: 2 in, 1 out]
                    n514 = String Length(string=w875) -> (length=w874:i32)
                    n515 = String Length(string=w870) -> (length=w873:i32)
                    n516 = Subtract(x=w884, y=w885) -> (x-y=w879:dbl)
                    n517 = Decrement(x=w874) -> (x-1=w868:i32)
                    n518 = Decrement(x=w873) -> (x-1=w867:i32)
                    n519 = Greater?(x=w868, y=w867) -> (0:w869:bool)
                    n520 = Select(t=w868, s=w869, f=w867) -> (s? t:f=w866:i32)
                    n521 = Number To Fractional String(number=w879, precision (6)=w866) -> (F-format string=w878:string)  [unwired: 2 in]
                    n522 = Concatenate Strings(w878, "/" ("string")) -> (w881:string)
                  }
                  frame 3 {
                    n523 = local read "String"() -> (w896:string)
                    n524 = local write "Numeric"(4.0 ("Numeric")) -> ()
                    n525 = Search/Split String(string=w896, search string/char (-)="*") -> (substring before match=w892:string, match + rest of string=w891:string)  [unwired: 1 in, 1 out]
                    n526 = Fract/Exp String To Number(string=w892) -> (number=w897:dbl)  [unwired: 3 in, 1 out]
                    n527 = Fract/Exp String To Number(string=w891, offset=1) -> (number=w898:dbl)  [unwired: 2 in, 1 out]
                    n528 = Multiply(x=w897, y=w898) -> (x*y=w889:dbl)
                    n529 = Format Into String(format string="%#.6f", w889) -> (resulting string=w888:string)  [unwired: 2 in, 1 out]
                    n530 = Concatenate Strings(w888, "/" ("string")) -> (w894:string)
                  }
                  frame 4 {
                    n531 = local read "String"() -> (w912:string)
                    n532 = Search/Split String(string=w912, search string/char (-)="/") -> (substring before match=w910:string, match + rest of string=w909:string)  [unwired: 1 in, 1 out]
                    n533 = local write "Numeric"(4.0 ("Numeric")) -> ()
                    n534 = Fract/Exp String To Number(string=w910) -> (number=w913:dbl)  [unwired: 3 in, 1 out]
                    n535 = Fract/Exp String To Number(string=w909, offset=1) -> (number=w906:dbl)  [unwired: 2 in, 1 out]
                    n536 = Equal To 0?(x=w906) -> (x = 0?=w908:bool)
                    n537 = Divide(x=w913, y=w906) -> (x/y=w902:dbl)
                    n538 = Format Into String(format string="%#.6f", w902) -> (resulting string=w901:string)  [unwired: 2 in, 1 out]
                    n539 = Concatenate Strings(w901, "/" ("string")) -> (w905:string)
                    n540 = Select(t="Error", s=w908, f=w905) -> (s? t:f=w904:string)
                  }
                  frame 5 {
                    n541 = local read "String"() -> (w917:string)
                    n542 = local write "Numeric"(4.0 ("Numeric")) -> ()
                    n543 = Concatenate Strings(w917, "/" ("string")) -> (w919:string)
                  }
                }
                n544 = local write "Boolean 30"(TRUE) -> ()
              }
            }
            n545 = local write "String"(w835) -> ()
          }
        }
      }
      event ".": Mouse Down {
        n546 = event-data() -> ()  [unwired: 1 in, 8 out]
        n547 = local read "Boolean 30"() -> (w922:bool)
        n548 = case shown="True" w922 {
          tunnel: ["Error" w924] -> w921
          frame True {
          }
          frame False {
            n549 = local read "String"() -> (w926:string)
            n550 = Concatenate Strings(w926, "." ("string")) -> (w924:string)
            n551 = local write "Boolean 30"(TRUE) -> ()
          }
        }
        n552 = local write "String"(w921) -> ()
      }
      event "+/-": Mouse Down {
        n553 = event-data() -> ()  [unwired: 1 in, 8 out]
        n554 = local read "Numeric"() -> (w928:dbl)
        n555 = case shown="0, Default" w928 {
          frame 0, Default {
            n556 = local read "String"() -> (w934:string)
            n557 = Fract/Exp String To Number(string=w934) -> (number=w933:dbl)  [unwired: 3 in, 1 out]
            n558 = Multiply(x=w933, y=-1.0) -> (x*y=w930:dbl)
            n559 = Format Into String(format string="%#.6f", w930) -> (resulting string=w929:string)  [unwired: 2 in, 1 out]
            n560 = local write "String"(w929) -> ()
          }
          frame 1 {
            n561 = local read "String"() -> (w944:string)
            n562 = Search/Split String(string=w944, search string/char (-)="+") -> (substring before match=w945:string, match + rest of string=w943:string)  [unwired: 1 in, 1 out]
            n563 = Fract/Exp String To Number(string=w943, offset=1) -> (number=w942:dbl)  [unwired: 2 in, 1 out]
            n564 = Multiply(x=w942, y=-1.0) -> (x*y=w936:dbl)
            n565 = Format Into String(format string="%#.6f", w936) -> (resulting string=w935:string)  [unwired: 2 in, 1 out]
            n566 = Concatenate Strings(w945, "+" ("string"), w935) -> (w946:string)
            n567 = local write "String"(w946) -> ()
          }
          frame 2 {
            n568 = local read "String"() -> (w956:string)
            n569 = Search/Split String(string=w956, search string/char (-)="-") -> (substring before match=w957:string, match + rest of string=w955:string)  [unwired: 1 in, 1 out]
            n570 = Fract/Exp String To Number(string=w955, offset=1) -> (number=w954:dbl)  [unwired: 2 in, 1 out]
            n571 = Multiply(x=w954, y=-1.0) -> (x*y=w948:dbl)
            n572 = Format Into String(format string="%#.6f", w948) -> (resulting string=w947:string)  [unwired: 2 in, 1 out]
            n573 = Concatenate Strings(w957, "-" ("string"), w947) -> (w958:string)
            n574 = local write "String"(w958) -> ()
          }
          frame 3 {
            n575 = local read "String"() -> (w969:string)
            n576 = Search/Split String(string=w969, search string/char (-)="*") -> (substring before match=w962:string, match + rest of string=w963:string)  [unwired: 1 in, 1 out]
            n577 = Fract/Exp String To Number(string=w963, offset=1) -> (number=w968:dbl)  [unwired: 2 in, 1 out]
            n578 = Multiply(x=w968, y=-1.0) -> (x*y=w960:dbl)
            n579 = Format Into String(format string="%#.6f", w960) -> (resulting string=w959:string)  [unwired: 2 in, 1 out]
            n580 = Concatenate Strings(w962, "*" ("string"), w959) -> (w970:string)
            n581 = local write "String"(w970) -> ()
          }
          frame 4 {
            n582 = local read "String"() -> (w980:string)
            n583 = Search/Split String(string=w980, search string/char (-)="/") -> (substring before match=w981:string, match + rest of string=w979:string)  [unwired: 1 in, 1 out]
            n584 = Fract/Exp String To Number(string=w979, offset=1) -> (number=w978:dbl)  [unwired: 2 in, 1 out]
            n585 = Multiply(x=w978, y=-1.0) -> (x*y=w972:dbl)
            n586 = Format Into String(format string="%#.6f", w972) -> (resulting string=w971:string)  [unwired: 2 in, 1 out]
            n587 = Concatenate Strings(w981, "/" ("string"), w971) -> (w982:string)
            n588 = local write "String"(w982) -> ()
          }
        }
      }
      event "=": Mouse Down {
        n589 = event-data() -> ()  [unwired: 1 in, 8 out]
        n590 = local read "Boolean 30"() -> (w984:bool)
        n591 = case shown="False" w984 {
          tunnel: ["Error" w987] -> w985
          frame True {
          }
          frame False {
            n592 = local read "Numeric"() -> (w990:dbl)
            n593 = case shown="1" w990 {
              tunnel: ["0" w1005 w1030 w1043 w1056 w1058] -> w987
              frame 0, Default {
                n594 = local write "Numeric"(-1.0 ("Numeric")) -> ()
              }
              frame 1 {
                n595 = local read "String"() -> (w1007:string)
                n596 = local write "Numeric"(-1.0 ("Numeric")) -> ()
                n597 = Search/Split String(string=w1007, search string/char (-)="+") -> (substring before match=w1014:string, match + rest of string=w1019:string)  [unwired: 1 in, 1 out]
                n598 = Search/Split String(string=w1014, search string/char (-)=".") -> (match + rest of string=w1016:string)  [unwired: 1 in, 2 out]
                n599 = Search/Split String(string=w1019, search string/char (-)=".") -> (match + rest of string=w1021:string)  [unwired: 1 in, 2 out]
                n600 = Fract/Exp String To Number(string=w1014) -> (number=w1012:dbl)  [unwired: 3 in, 1 out]
                n601 = Fract/Exp String To Number(string=w1019, offset=1) -> (number=w1011:dbl)  [unwired: 2 in, 1 out]
                n602 = String Length(string=w1016) -> (length=w1017:i32)
                n603 = String Length(string=w1021) -> (length=w1018:i32)
                n604 = Add(x=w1012, y=w1011) -> (x+y=w1013:dbl)
                n605 = Decrement(x=w1017) -> (x-1=w1023:i32)
                n606 = Decrement(x=w1018) -> (x-1=w1024:i32)
                n607 = Greater?(x=w1023, y=w1024) -> (0:w1022:bool)
                n608 = Select(t=w1023, s=w1022, f=w1024) -> (s? t:f=w1025:i32)
                n609 = Number To Fractional String(number=w1013, precision (6)=w1025) -> (F-format string=w1008:string)  [unwired: 2 in]
                n610 = Concatenate Strings(w1007, "=" ("string"), w1008) -> (w1005:string)
              }
              frame 3 {
                n611 = local read "String"() -> (w1032:string)
                n612 = local write "Numeric"(-1.0 ("Numeric")) -> ()
                n613 = Search/Split String(string=w1032, search string/char (-)="*") -> (substring before match=w1037:string, match + rest of string=w1038:string)  [unwired: 1 in, 1 out]
                n614 = Fract/Exp String To Number(string=w1037) -> (number=w1036:dbl)  [unwired: 3 in, 1 out]
                n615 = Fract/Exp String To Number(string=w1038, offset=1) -> (number=w1035:dbl)  [unwired: 2 in, 1 out]
                n616 = Multiply(x=w1036, y=w1035) -> (x*y=w1028:dbl)
                n617 = Format Into String(format string="%#.6f", w1028) -> (resulting string=w1027:string)  [unwired: 2 in, 1 out]
                n618 = Concatenate Strings(w1032, "=" ("string"), w1027) -> (w1030:string)
              }
              frame 4 {
                n619 = local read "String"() -> (w1049:string)
                n620 = local write "Numeric"(-1.0 ("Numeric")) -> ()
                n621 = Search/Split String(string=w1049, search string/char (-)="/") -> (substring before match=w1051:string, match + rest of string=w1050:string)  [unwired: 1 in, 1 out]
                n622 = Fract/Exp String To Number(string=w1051) -> (number=w1052:dbl)  [unwired: 3 in, 1 out]
                n623 = Fract/Exp String To Number(string=w1050, offset=1) -> (number=w1046:dbl)  [unwired: 2 in, 1 out]
                n624 = Equal To 0?(x=w1046) -> (x = 0?=w1047:bool)
                n625 = Divide(x=w1052, y=w1046) -> (x/y=w1041:dbl)
                n626 = Format Into String(format string="%#.6f", w1041) -> (resulting string=w1040:string)  [unwired: 2 in, 1 out]
                n627 = Concatenate Strings(w1049, "=" ("string"), w1040) -> (w1045:string)
                n628 = Select(t="Error", s=w1047, f=w1045) -> (s? t:f=w1043:string)
              }
              frame 5 {
                n629 = local read "String"() -> (w1056:string)
                n630 = local write "Numeric"(-1.0 ("Numeric")) -> ()
              }
              frame 2 {
                n631 = local read "String"() -> (w1060:string)
                n632 = local write "Numeric"(-1.0 ("Numeric")) -> ()
                n633 = Search/Split String(string=w1060, search string/char (-)="-") -> (substring before match=w1067:string, match + rest of string=w1072:string)  [unwired: 1 in, 1 out]
                n634 = Search/Split String(string=w1067, search string/char (-)=".") -> (match + rest of string=w1069:string)  [unwired: 1 in, 2 out]
                n635 = Search/Split String(string=w1072, search string/char (-)=".") -> (match + rest of string=w1074:string)  [unwired: 1 in, 2 out]
                n636 = Fract/Exp String To Number(string=w1067) -> (number=w1065:dbl)  [unwired: 3 in, 1 out]
                n637 = Fract/Exp String To Number(string=w1072, offset=1) -> (number=w1064:dbl)  [unwired: 2 in, 1 out]
                n638 = String Length(string=w1069) -> (length=w1070:i32)
                n639 = String Length(string=w1074) -> (length=w1071:i32)
                n640 = Subtract(x=w1065, y=w1064) -> (x-y=w1066:dbl)
                n641 = Decrement(x=w1070) -> (x-1=w1076:i32)
                n642 = Decrement(x=w1071) -> (x-1=w1077:i32)
                n643 = Greater?(x=w1076, y=w1077) -> (0:w1075:bool)
                n644 = Select(t=w1076, s=w1075, f=w1077) -> (s? t:f=w1078:i32)
                n645 = Number To Fractional String(number=w1066, precision (6)=w1078) -> (F-format string=w1061:string)  [unwired: 2 in]
                n646 = Concatenate Strings(w1060, "=" ("string"), w1061) -> (w1058:string)
              }
            }
            n647 = local write "Boolean 30"(TRUE) -> ()
            n648 = case shown="True" "Boolean" {
              tunnel: w987 -> [w992 w1002]
              frame False {
                n649 = Search/Split String(string=w992, search string/char (-)="=") -> (match + rest of string=w996:string)  [unwired: 1 in, 2 out]
                n650 = local write "Boolean"(TRUE) -> ()
                n651 = Fract/Exp String To Number(string=w996, offset=1) -> (number=→"two":dbl)  [unwired: 2 in, 1 out]
              }
              frame True {
                n652 = Search/Split String(string=w1002, search string/char (-)="=") -> (match + rest of string=w1000:string)  [unwired: 1 in, 2 out]
                n653 = local write "Boolean"(FALSE ("Boolean")) -> ()
                n654 = Fract/Exp String To Number(string=w1000, offset=1) -> (number=→"History one":dbl)  [unwired: 2 in, 1 out]
              }
            }
          }
        }
        n655 = local write "String"(w985) -> ()
        "Boolean 36" <- TRUE ("Boolean 36")
      }
      event ")": Mouse Down {
        n656 = event-data() -> ()  [unwired: 1 in, 8 out]
        n657 = case shown="False" "Boolean 35" {
          frame True {
            n658 = local write "String"("Error") -> ()
          }
          frame False {
            n659 = local read "String"() -> (w1090:string)
            n660 = local read "String"() -> (w1087:string)
            n661 = Equal?(x=w1087, y="0") -> (x = y?=w1088:bool)
            n662 = Concatenate Strings(w1090, ")" ("string")) -> (w1084:string)
            n663 = Select(t=")" ("string"), s=w1088, f=w1084) -> (s? t:f=w1085:string)
            n664 = local write "String"(w1085) -> ()
            n665 = local write "Boolean 35"(TRUE) -> ()
          }
        }
      }
      event "(": Mouse Down {
        n666 = event-data() -> ()  [unwired: 1 in, 8 out]
        n667 = local read "Boolean 35"() -> (w1091:bool)
        n668 = case shown="False" w1091 {
          frame True {
            n669 = local write "String"("Error") -> ()
          }
          frame False {
            n670 = local read "String"() -> (w1101:string)
            n671 = local read "String"() -> (w1098:string)
            n672 = Equal?(x=w1098, y="0") -> (x = y?=w1099:bool)
            n673 = Concatenate Strings(w1101, "(" ("string")) -> (w1095:string)
            n674 = Select(t="(" ("string"), s=w1099, f=w1095) -> (s? t:f=w1096:string)
            n675 = local write "String"(w1096) -> ()
            n676 = local write "Boolean 35"(TRUE) -> ()
          }
        }
      }
      event "C": Mouse Down {
        n677 = event-data() -> ()  [unwired: 1 in, 8 out]
        n678 = local read "String"() -> (w1109:string)
        n679 = Two Button Dialog(message="是否確認清除", 1:"否" ("F button name (\"Cancel\")"), 2:"是" ("T button name (\"OK\")")) -> (T button?=w1106:bool)
        n680 = Equal?(x=w1106, y=TRUE) -> (x = y?=w1105:bool)
        n681 = Select(t="0" ("String"), s=w1105, f=w1109) -> (s? t:f=w1108:string)
        n682 = local write "String"(w1108) -> ()
        n683 = Select(t=FALSE ("Boolean 35"), s=w1105, f=TRUE) -> (s? t:f=w1102:bool)
        n684 = local write "Boolean 36"(w1102) -> ()
      }
      event "Backspace": Mouse Down {
        n685 = event-data() -> ()  [unwired: 1 in, 8 out]
        n686 = local read "String"() -> (w1117:string)
        n687 = String To Byte Array(string=w1117) -> (unsigned byte array=w1116:u8[])
        n688 = Delete From Array(array=w1116) -> (array with subset deleted=w1115:u8[])  [unwired: 2 in, 1 out]
        n689 = Byte Array To String(unsigned byte array=w1115) -> (string=w1114:string)
        n690 = local write "String"(w1114) -> ()
      }
    }
    n691 = local read "Boolean"() -> (w9:bool)
    n692 = case shown="False" w9 {
      frame False {
        n693 = local read "History one"() -> (w51:dbl)
        n694 = Quotient & Remainder(x=w51, y=10.0) -> (x-y*floor(x/y)=w49:dbl, floor(x/y)=w38:dbl)
        n695 = Quotient & Remainder(x=w38, y=10.0) -> (x-y*floor(x/y)=w36:dbl, floor(x/y)=w30:dbl)
        n696 = case shown="1" w36 {
          tunnel: [w90 w92 w94 w96 w98 w100 w102 w105 w106 w107] -> w43
          tunnel: [w90 w92 w95 w97 w99 w100 w102 w104 w106 w107] -> w42
          tunnel: [FALSE w92 w94 w96 w99 w100 w102 w104 w106 w107] -> w41
          tunnel: [w90 w93 w94 w96 w99 w101 FALSE w105 w106 w107] -> w40
          tunnel: [w90 w92 w94 w97 w98 w101 w102 w104 w106 FALSE] -> w39
          tunnel: [w90 w93 w95 w96 w99 w100 w102 w105 w106 w107] -> w12
          tunnel: [w90 w92 w94 w96 w98 w100 w102 w104 w106 w107] -> w13
          frame 0, Default {
            w90 = TRUE
          }
          frame 1 {
            w92 = FALSE
            w93 = TRUE
          }
          frame 2 {
            w95 = FALSE
            w94 = TRUE
          }
          frame 3 {
            w97 = FALSE
            w96 = TRUE
          }
          frame 4 {
            w99 = TRUE
            w98 = FALSE
          }
          frame 5 {
            w101 = FALSE
            w100 = TRUE
          }
          frame 6 {
            w102 = TRUE
          }
          frame 7 {
            w104 = FALSE
            w105 = TRUE
          }
          frame 8 {
            w106 = TRUE
          }
          frame 9 {
            w107 = TRUE
          }
        }
        "Boolean 16" <- w43
        "Boolean 17" <- w13
        "Boolean 18" <- w41
        "Boolean 19" <- w40
        "Boolean 20" <- w12
        "Boolean 21" <- w42
        "Boolean 22" <- w39
        n697 = case shown="4" w49 {
          tunnel: [w109 w111 w113 w115 w117 w119 w121 w124 w125 w126] -> w48
          tunnel: [w109 w111 w114 w116 w118 w119 w121 w123 w125 w126] -> w47
          tunnel: [FALSE w111 w113 w115 w118 w119 w121 w123 w125 w126] -> w46
          tunnel: [w109 w112 w113 w115 w118 w120 FALSE w124 w125 w126] -> w45
          tunnel: [w109 w111 w113 w116 w117 w120 w121 w123 w125 FALSE] -> w44
          tunnel: [w109 w112 w114 w115 w118 w119 w121 w124 w125 w126] -> w14
          tunnel: [w109 w111 w113 w115 w117 w119 w121 w123 w125 w126] -> w15
          frame 0, Default {
            w109 = TRUE
          }
          frame 1 {
            w111 = FALSE
            w112 = TRUE
          }
          frame 2 {
            w114 = FALSE
            w113 = TRUE
          }
          frame 3 {
            w116 = FALSE
            w115 = TRUE
          }
          frame 4 {
            w118 = TRUE
            w117 = FALSE
          }
          frame 5 {
            w120 = FALSE
            w119 = TRUE
          }
          frame 6 {
            w121 = TRUE
          }
          frame 7 {
            w123 = FALSE
            w124 = TRUE
          }
          frame 8 {
            w125 = TRUE
          }
          frame 9 {
            w126 = TRUE
          }
        }
        "Boolean 23" <- w48
        "Boolean 28" <- w47
        "Boolean 25" <- w46
        "Boolean 26" <- w45
        "Boolean 29" <- w44
        "Boolean 24" <- w15
        "Boolean 27" <- w14
        n698 = Quotient & Remainder(x=w30, y=10.0) -> (x-y*floor(x/y)=w28:dbl, floor(x/y)=w27:dbl)
        n699 = Quotient & Remainder(x=w27, y=10.0) -> (x-y*floor(x/y)=w25:dbl)  [unwired: 1 out]
        n700 = case shown="1" w28 {
          tunnel: [w71 w73 w75 w77 w79 w81 w83 w86 w87 w88] -> w35
          tunnel: [w71 w73 w76 w78 w80 w81 w83 w85 w87 w88] -> w34
          tunnel: [FALSE w73 w75 w77 w80 w81 w83 w85 w87 w88] -> w33
          tunnel: [w71 w74 w75 w77 w80 w82 FALSE w86 w87 w88] -> w32
          tunnel: [w71 w73 w75 w78 w79 w82 w83 w85 w87 FALSE] -> w31
          tunnel: [w71 w74 w76 w77 w80 w81 w83 w86 w87 w88] -> w16
          tunnel: [w71 w73 w75 w77 w79 w81 w83 w85 w87 w88] -> w17
          frame 0, Default {
            w71 = TRUE
          }
          frame 1 {
            w73 = FALSE
            w74 = TRUE
          }
          frame 2 {
            w76 = FALSE
            w75 = TRUE
          }
          frame 3 {
            w78 = FALSE
            w77 = TRUE
          }
          frame 4 {
            w80 = TRUE
            w79 = FALSE
          }
          frame 5 {
            w82 = FALSE
            w81 = TRUE
          }
          frame 6 {
            w83 = TRUE
          }
          frame 7 {
            w85 = FALSE
            w86 = TRUE
          }
          frame 8 {
            w87 = TRUE
          }
          frame 9 {
            w88 = TRUE
          }
        }
        "Boolean 9" <- w35
        "Boolean 10" <- w17
        "Boolean 11" <- w33
        "Boolean 12" <- w32
        "Boolean 13" <- w16
        "Boolean 14" <- w34
        "Boolean 15" <- w31
        n701 = case shown="0, Default" w25 {
          tunnel: [w52 w54 w56 w58 w60 w62 w64 w67 w68 w69] -> w24
          tunnel: [w52 w54 w57 w59 w61 w62 w64 w66 w68 w69] -> w23
          tunnel: [FALSE w54 w56 w58 w61 w62 w64 w66 w68 w69] -> w22
          tunnel: [w52 w55 w56 w58 w61 w63 FALSE w67 w68 w69] -> w21
          tunnel: [w52 w54 w56 w59 w60 w63 w64 w66 w68 FALSE] -> w20
          tunnel: [w52 w55 w57 w58 w61 w62 w64 w67 w68 w69] -> w19
          tunnel: [w52 w54 w56 w58 w60 w62 w64 w66 w68 w69] -> w18
          frame 0, Default {
            w52 = TRUE
          }
          frame 1 {
            w54 = FALSE
            w55 = TRUE
          }
          frame 2 {
            w57 = FALSE
            w56 = TRUE
          }
          frame 3 {
            w59 = FALSE
            w58 = TRUE
          }
          frame 4 {
            w61 = TRUE
            w60 = FALSE
          }
          frame 5 {
            w63 = FALSE
            w62 = TRUE
          }
          frame 6 {
            w64 = TRUE
          }
          frame 7 {
            w66 = FALSE
            w67 = TRUE
          }
          frame 8 {
            w68 = TRUE
          }
          frame 9 {
            w69 = TRUE
          }
        }
        "Boolean 4" <- w22
        "Boolean 2" <- w24
        "Boolean 3" <- w18
        "Boolean 5" <- w21
        "Boolean 8" <- w20
        "Boolean 6" <- w19
        "Boolean 7" <- w23
      }
      frame True {
        n702 = local read "two"() -> (w128:dbl)
        n703 = Quotient & Remainder(x=w128, y=10.0) -> (x-y*floor(x/y)=w166:dbl, floor(x/y)=w165:dbl)
        n704 = Quotient & Remainder(x=w165, y=10.0) -> (x-y*floor(x/y)=w163:dbl, floor(x/y)=w131:dbl)
        n705 = case shown="0, Default" w163 {
          tunnel: [w206 w208 w210 w212 w214 w216 w218 w221 w222 w223] -> w152
          tunnel: [w206 w208 w211 w213 w215 w216 w218 w220 w222 w223] -> w151
          tunnel: [FALSE w208 w210 w212 w215 w216 w218 w220 w222 w223] -> w150
          tunnel: [w206 w209 w210 w212 w215 w217 FALSE w221 w222 w223] -> w149
          tunnel: [w206 w208 w210 w213 w214 w217 w218 w220 w222 FALSE] -> w148
          tunnel: [w206 w209 w211 w212 w215 w216 w218 w221 w222 w223] -> w147
          tunnel: [w206 w208 w210 w212 w214 w216 w218 w220 w222 w223] -> w146
          frame 0, Default {
            w206 = TRUE
          }
          frame 1 {
            w208 = FALSE
            w209 = TRUE
          }
          frame 2 {
            w211 = FALSE
            w210 = TRUE
          }
          frame 3 {
            w213 = FALSE
            w212 = TRUE
          }
          frame 4 {
            w215 = TRUE
            w214 = FALSE
          }
          frame 5 {
            w217 = FALSE
            w216 = TRUE
          }
          frame 6 {
            w218 = TRUE
          }
          frame 7 {
            w220 = FALSE
            w221 = TRUE
          }
          frame 8 {
            w222 = TRUE
          }
          frame 9 {
            w223 = TRUE
          }
        }
        n706 = case shown="0, Default" w166 {
          tunnel: [w225 w227 w229 w231 w233 w235 w237 w240 w241 w242] -> w158
          tunnel: [w225 w227 w230 w232 w234 w235 w237 w239 w241 w242] -> w157
          tunnel: [FALSE w227 w229 w231 w234 w235 w237 w239 w241 w242] -> w156
          tunnel: [w225 w228 w229 w231 w234 w236 FALSE w240 w241 w242] -> w155
          tunnel: [w225 w227 w229 w232 w233 w236 w237 w239 w241 FALSE] -> w154
          tunnel: [w225 w228 w230 w231 w234 w235 w237 w240 w241 w242] -> w153
          tunnel: [w225 w227 w229 w231 w233 w235 w237 w239 w241 w242] -> w129
          frame 0, Default {
            w225 = TRUE
          }
          frame 1 {
            w227 = FALSE
            w228 = TRUE
          }
          frame 2 {
            w230 = FALSE
            w229 = TRUE
          }
          frame 3 {
            w232 = FALSE
            w231 = TRUE
          }
          frame 4 {
            w234 = TRUE
            w233 = FALSE
          }
          frame 5 {
            w236 = FALSE
            w235 = TRUE
          }
          frame 6 {
            w237 = TRUE
          }
          frame 7 {
            w239 = FALSE
            w240 = TRUE
          }
          frame 8 {
            w241 = TRUE
          }
          frame 9 {
            w242 = TRUE
          }
        }
        n707 = local write "Boolean 23"(w158) -> ()
        n708 = local write "Boolean 28"(w157) -> ()
        n709 = local write "Boolean 25"(w156) -> ()
        n710 = local write "Boolean 26"(w155) -> ()
        n711 = local write "Boolean 29"(w154) -> ()
        n712 = local write "Boolean 24"(w129) -> ()
        n713 = local write "Boolean 27"(w153) -> ()
        n714 = local write "Boolean 16"(w152) -> ()
        n715 = local write "Boolean 21"(w151) -> ()
        n716 = local write "Boolean 18"(w150) -> ()
        n717 = local write "Boolean 19"(w149) -> ()
        n718 = local write "Boolean 22"(w148) -> ()
        n719 = local write "Boolean 17"(w146) -> ()
        n720 = local write "Boolean 20"(w147) -> ()
        n721 = Quotient & Remainder(x=w131, y=10.0) -> (x-y*floor(x/y)=w162:dbl, floor(x/y)=w161:dbl)
        n722 = Quotient & Remainder(x=w161, y=10.0) -> (x-y*floor(x/y)=w159:dbl)  [unwired: 1 out]
        n723 = case shown="0, Default" w162 {
          tunnel: [w187 w189 w191 w193 w195 w197 w199 w202 w203 w204] -> w145
          tunnel: [w187 w189 w192 w194 w196 w197 w199 w201 w203 w204] -> w144
          tunnel: [FALSE w189 w191 w193 w196 w197 w199 w201 w203 w204] -> w143
          tunnel: [w187 w190 w191 w193 w196 w198 FALSE w202 w203 w204] -> w142
          tunnel: [w187 w189 w191 w194 w195 w198 w199 w201 w203 FALSE] -> w141
          tunnel: [w187 w190 w192 w193 w196 w197 w199 w202 w203 w204] -> w140
          tunnel: [w187 w189 w191 w193 w195 w197 w199 w201 w203 w204] -> w139
          frame 0, Default {
            w187 = TRUE
          }
          frame 1 {
            w189 = FALSE
            w190 = TRUE
          }
          frame 2 {
            w192 = FALSE
            w191 = TRUE
          }
          frame 3 {
            w194 = FALSE
            w193 = TRUE
          }
          frame 4 {
            w196 = TRUE
            w195 = FALSE
          }
          frame 5 {
            w198 = FALSE
            w197 = TRUE
          }
          frame 6 {
            w199 = TRUE
          }
          frame 7 {
            w201 = FALSE
            w202 = TRUE
          }
          frame 8 {
            w203 = TRUE
          }
          frame 9 {
            w204 = TRUE
          }
        }
        n724 = case shown="0, Default" w159 {
          tunnel: [w168 w170 w172 w174 w176 w178 w180 w183 w184 w185] -> w138
          tunnel: [w168 w170 w173 w175 w177 w178 w180 w182 w184 w185] -> w137
          tunnel: [FALSE w170 w172 w174 w177 w178 w180 w182 w184 w185] -> w136
          tunnel: [w168 w171 w172 w174 w177 w179 FALSE w183 w184 w185] -> w135
          tunnel: [w168 w170 w172 w175 w176 w179 w180 w182 w184 FALSE] -> w134
          tunnel: [w168 w171 w173 w174 w177 w178 w180 w183 w184 w185] -> w133
          tunnel: [w168 w170 w172 w174 w176 w178 w180 w182 w184 w185] -> w132
          frame 0, Default {
            w168 = TRUE
          }
          frame 1 {
            w170 = FALSE
            w171 = TRUE
          }
          frame 2 {
            w173 = FALSE
            w172 = TRUE
          }
          frame 3 {
            w175 = FALSE
            w174 = TRUE
          }
          frame 4 {
            w177 = TRUE
            w176 = FALSE
          }
          frame 5 {
            w179 = FALSE
            w178 = TRUE
          }
          frame 6 {
            w180 = TRUE
          }
          frame 7 {
            w182 = FALSE
            w183 = TRUE
          }
          frame 8 {
            w184 = TRUE
          }
          frame 9 {
            w185 = TRUE
          }
        }
        n725 = local write "Boolean 14"(w144) -> ()
        n726 = local write "Boolean 9"(w145) -> ()
        n727 = local write "Boolean 11"(w143) -> ()
        n728 = local write "Boolean 12"(w142) -> ()
        n729 = local write "Boolean 15"(w141) -> ()
        n730 = local write "Boolean 10"(w139) -> ()
        n731 = local write "Boolean 13"(w140) -> ()
        n732 = local write "Boolean 2"(w138) -> ()
        n733 = local write "Boolean 7"(w137) -> ()
        n734 = local write "Boolean 4"(w136) -> ()
        n735 = local write "Boolean 5"(w135) -> ()
        n736 = local write "Boolean 8"(w134) -> ()
        n737 = local write "Boolean 3"(w132) -> ()
        n738 = local write "Boolean 6"(w133) -> ()
      }
    }
  }
  n739 = while {
    i -> [w1120]
    stop <- w1119 stop-if-true
    n740 = event shown="[0] Timeout" {
      selector: _ -> [_ _]
      dyn-events: _ -> [_ _]
      timeout: 1000.0 -> [_ _]
      tunnel: w1120 -> [w1121 _]
      tunnel: [_ TRUE] -> w1119
      event Timeout {
        n741 = event-data() -> ()  [unwired: 1 in, 3 out]
        n742 = Quotient & Remainder(x=w1121, y=u32 60) -> (x-y*floor(x/y)=w1140:u32, floor(x/y)=w1137:u32)
        n743 = Get Date/Time String() -> (time string=w1123:string)  [unwired: 3 in, 1 out]
        n744 = Quotient & Remainder(x=w1137, y=u32 60) -> (x-y*floor(x/y)=w1135:u32, floor(x/y)=w1132:u32)
        n745 = Number To Fractional String(number=w1140, precision (6)=i16 0) -> (F-format string=w1128:string)  [unwired: 2 in]
        n746 = Number To Fractional String(number=w1135, precision (6)=i16 0) -> (F-format string=w1129:string)  [unwired: 2 in]
        n747 = Number To Fractional String(number=w1132, precision (6)=i16 0) -> (F-format string=w1127:string)  [unwired: 2 in]
        n748 = Concatenate Strings("現在時間:" ("string"), w1123, "\n" ("string"), "已花時間:" ("string"), w1127, ":" ("string"), w1129, ":" ("string"), w1128) -> (→"String 2":string)
      }
      event "stop": Mouse Down {
        n749 = event-data() -> ()  [unwired: 1 in, 6 out]
      }
    }
  }
  "String" <- "0" ("String")
  "Numeric" <- -1.0 ("Numeric")
